vi "Activate Message View.vi"(8 "error in (no error)":errorcluster, 11 "Main In":refnum<class "Main.lvclass">) -> (0 "error out":errorcluster, 2 "VI Ref":refnum<vi>, 3 "Main Out":refnum<class "Main.lvclass">)   [LabVIEW 2020, in "Main.lvclass"]
uses:
  Main.lvclass
  Messages Composite View/Messages Composite View.lvclass
  C:/Users/anton/Documents/GitHub/triarc-debugger/source/Debug View/Debug View.lvclass
  Debug View/Debug View.lvclass/Debug View.ctl
  Debugger/Debugger.lvclass
  C:/Users/anton/Documents/GitHub/triarc-debugger/source/Process/Debug Process.lvclass
  Debug View/Debug View.lvclass
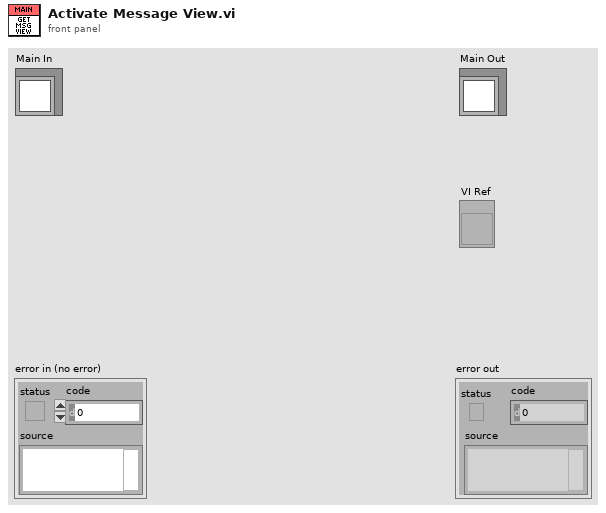
[diagram p1: front panel]
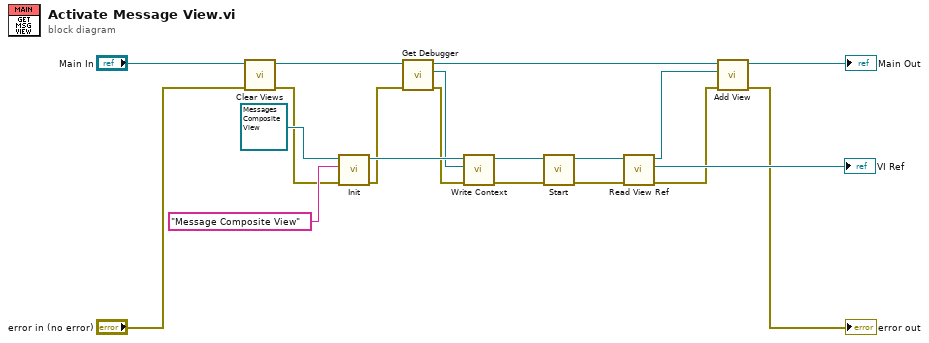
[diagram p0: block diagram]
diagram:
  n1 = call "Clear Views.vi"("error in (no error)"="error in (no error)", "Main In"="Main In") -> ("error out"=w1:errorcluster, "Main Out"=w13:refnum<class "Main.lvclass">)  [unwired: 8 in]
  n2 = call-dynamic "Init.vi"("error in (no error)"=w1, "Name"="Message Composite View", "Debug View In"=refnum<class "Messages Composite View.lvclass"> refnum ("Messages Composite View.lvclass")) -> ("error out"=w11:errorcluster, "Debug View Out"=w15:refnum<class "Messages Composite View.lvclass">)  [unwired: 7 in]
  n3 = call "Get Debugger.vi"("error in (no error)"=w11, "Main In"=w13) -> ("error out"=w10:errorcluster, "Debugger.lvclass"=w12:refnum<class "Debugger.lvclass">, "Main Out"=w5:refnum<class "Main.lvclass">)  [unwired: 7 in]
  n4 = call "Write Context.vi"("error in (no error)"=w10, "Debug Process.lvclass"=w12, "Debug View In"=w15) -> ("error out"=w17:errorcluster, "Debug View Out"=w16:refnum<class "Messages Composite View.lvclass">)  [unwired: 7 in]
  n5 = call "Start.vi"("error in (no error)"=w17, "Debug View In"=w16) -> ("error out"=w8:errorcluster, "Debug View Out"=w9:refnum<class "Messages Composite View.lvclass">)  [unwired: 8 in]
  n6 = call "Read View Ref.vi"("error in (no error)"=w8, "Debug View In"=w9) -> ("error out"=w7:errorcluster, "View Ref"=→"VI Ref":refnum<vi>, "Debug View Out"=w3:refnum<class "Messages Composite View.lvclass">)  [unwired: 7 in]
  n7 = call "Add View.vi"("error in (no error)"=w7, "Debug Process"=w3, "Main In"=w5) -> ("error out"=→"error out":errorcluster, "Main Out"=→"Main Out":refnum<class "Main.lvclass">)  [unwired: 7 in]
